vi "Set Data In.vi"(8 "error in (no error)":errorcluster, 11 "DataIn":T1) -> (0 "error out":errorcluster)   [LabVIEW 2017]
doc: "This VI writes the data received from the MLC to a FGV"
uses:
  TypeDefs/dataIn.ctl
  FGVs/TypeDefs/DataFGVControl.ctl
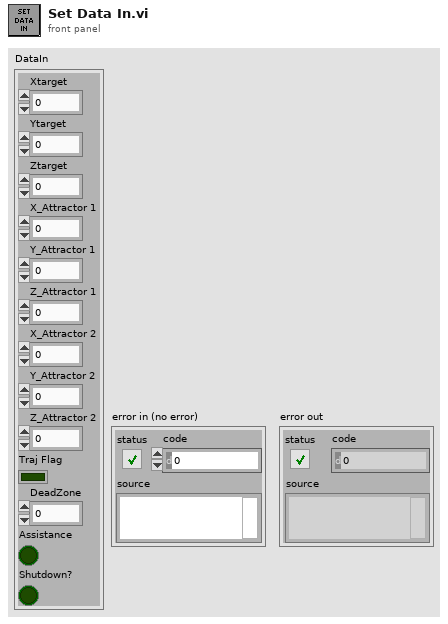
[diagram p1: front panel]
types:
  T1 = typedef "dataIn.ctl" = cluster{"Xtarget":dbl, "Ytarget":dbl, "Ztarget":dbl, "X_Attractor 1":dbl, "Y_Attractor 1":dbl, "Z_Attractor 1":dbl, "X_Attractor 2":dbl, "Y_Attractor 2":dbl, "Z_Attractor 2":dbl, "Traj Flag":bool, "DeadZone":dbl, "Assistance":bool, "Shutdown?":bool}
  T2 = typedef "DataFGVControl.ctl" = enum16{"Set Data", "Get Data"}
  T3 = typedef "allData.ctl" = cluster{"DataOut":T4, "DataIn":T1}
  T4 = typedef "dataOut.ctl" = cluster{"X0pos":dbl, "Y0pos":dbl, "Z0pos":dbl, "Fx":dbl, "Fy":dbl, "Fz":dbl, "Encoder1":i32, "Encoder2":i32, "Pot1":dbl, "Pot2":dbl, "Theta0":dbl, "Theta1":dbl, "X1pos":dbl, "Y1pos":dbl, "Z1pos":dbl, "X2pos":dbl, "Y2pos":dbl, "Z2pos":dbl, "ErrorOccurred":bool}
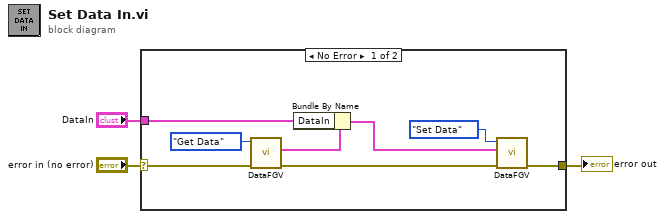
[diagram p0: block diagram]
diagram:
  n1 = case shown="No Error" "error in (no error)" {
    selector: "error in (no error)" -> [w10 w12]
    tunnel: [w7 w12] -> w2
    tunnel: "DataIn" -> [w5 _]
    frame No Error {
      n2 = call "DataFGV.vi"("error in (no error)"=w10, "Command"=DataFGVControl."Get Data") -> ("error out"=w9:errorcluster, "AllData out"=w6:T3)  [unwired: 8 in]
      n3 = Bundle By Name(cluster=w6, "DataIn"=w5) -> (w4:T3)
      n4 = call "DataFGV.vi"("error in (no error)"=w9, "AllData in"=w4, "Command"=DataFGVControl."Set Data") -> ("error out"=w7:errorcluster)  [unwired: 7 in, 1 out]
    }
    frame Error {
    }
  }
  "error out" <- w2
